vi "GUNSC_LibEnable.vi"(8 "error in (no error)":errorcluster, 10 "flag":bool) -> (0 "error out":errorcluster, 2 "return value":i32)   [LabVIEW 2016]
uses:
  public/c/lib/libunsc.so
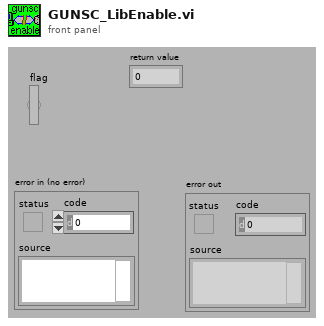
[diagram p1: front panel]
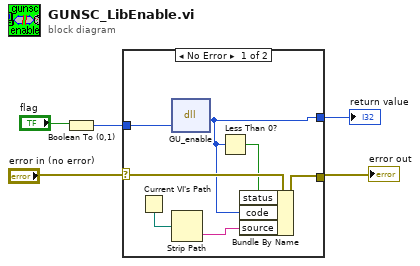
[diagram p0: block diagram]
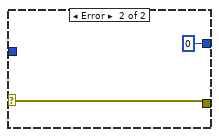
[diagram p2: hidden frame]
diagram:
  n1 = Boolean To (0,1)(Boolean="flag") -> (0, 1=w1:i16)
  n2 = case shown="No Error" "error in (no error)" {
    selector: "error in (no error)" -> [w11 w14]
    tunnel: w1 -> [w12 _]
    tunnel: [w9 0] -> w4
    tunnel: [w6 w14] -> w2
    frame No Error {
      n3 = Current VI's Path() -> (path=w8:path)
      n4 = dll-call lib="home/simager/panview/PAN/Modules/GUNSC/public/c/lib/libunsc.so" fn="GU_enable"("flag"=w12) -> ("return type"=w9:i32)  [unwired: 3 in, 3 out]
      n5 = Strip Path(path=w8) -> (name=w7:string)  [unwired: 1 out]
      n6 = Less Than 0?(x=w9) -> (x < 0?=w10:bool)
      n7 = Bundle By Name(cluster=w11, "status"=w10, "code"=w9, "source"=w7) -> (w6:errorcluster)
    }
    frame Error {
    }
  }
  "return value" <- w4
  "error out" <- w2
